vi "DSF.Execution.Builder.Get Framework Cache.vi"(8 "error in (no error)":errorcluster, 11 "Builder in":refnum<class "DSF.Execution.Builder.lvclass">) -> (0 "error out":errorcluster, 2 "Framework Cache":refnum<class "DSF.Engine.Memory.Cache.Framework.lvclass">, 3 "Builder out":refnum<class "DSF.Execution.Builder.lvclass">)   [LabVIEW 2016, in "DSF.Engine.lvlib" / "DSF.Execution.Builder.lvclass"]
uses:
  DSF.Execution.Builder.lvclass
  Memory.Cache/DSF.Engine.Memory.Cache.Framework.lvclass
  DSF.Execution.Builder.lvclass/DSF.Execution.Builder.ctl
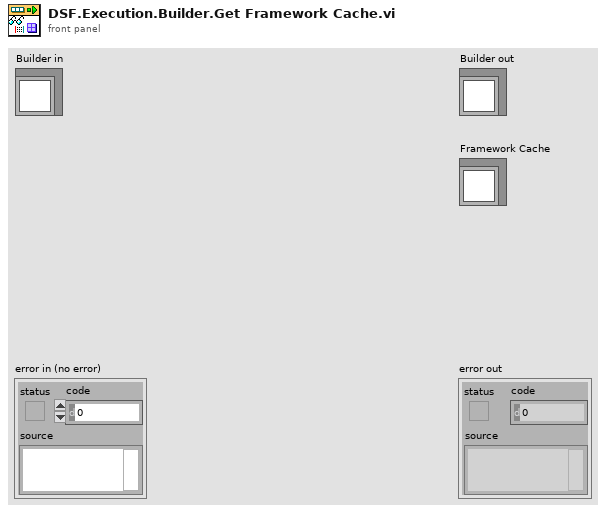
[diagram p1: front panel]
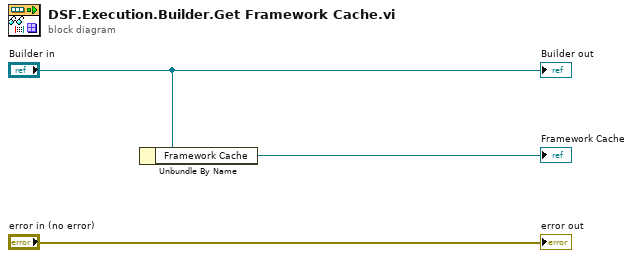
[diagram p0: block diagram]
diagram:
  n1 = Unbundle By Name("Builder in") -> ("Framework Cache"=→"Framework Cache":refnum<class "DSF.Engine.Memory.Cache.Framework.lvclass">)
  "error out" <- "error in (no error)"
  "Builder out" <- "Builder in"
